vi "TDC_preselectSingleStop.vi"(8 "Error In":errorcluster, 11 "Single Stop":bool) -> (0 "Error Out":errorcluster)   [LabVIEW 2011]
uses:
  tdcbase.dll
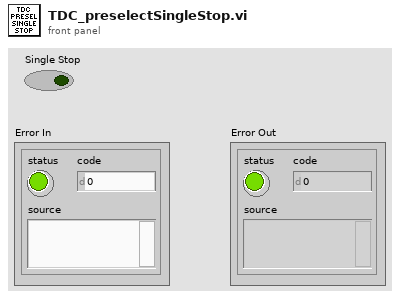
[diagram p1: front panel]
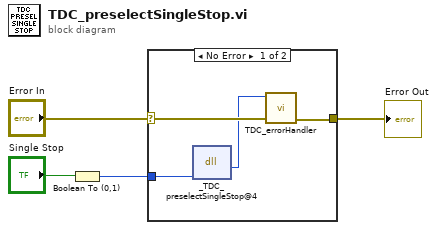
[diagram p0: block diagram]
diagram:
  n1 = Boolean To (0,1)(Boolean="Single Stop") -> (0, 1=w1:i16)
  n2 = case shown="No Error" "Error In" {
    selector: "Error In" -> [w8 w9]
    tunnel: [w6 w9] -> w3
    tunnel: w1 -> [w5 _]
    frame No Error {
      n3 = dll-call lib="X:/tdcbase.dll" fn="_TDC_preselectSingleStop@4"("singleStop"=w5) -> ("return type"=w7:i32)  [unwired: 4 in, 2 out]
      n4 = call "TDC_errorHandler.vi"("Error In"=w8, "TDC Return Code"=w7) -> ("Error Out"=w6:errorcluster)  [unwired: 9 in]
    }
    frame Error {
    }
  }
  "Error Out" <- w3
